vi "BUILD_uninstall tag bus.vi"() -> ()   [LabVIEW 2013]
panel:
  out "error out":errorcluster
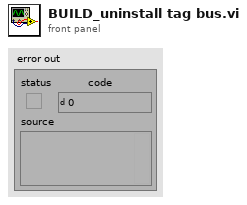
[diagram p1: front panel]
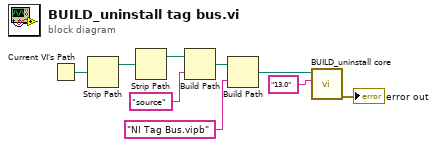
[diagram p0: block diagram]
diagram:
  n1 = Current VI's Path() -> (path=w9:path)
  n2 = Strip Path(path=w9) -> (stripped path=w8:path)  [unwired: 1 out]
  n3 = Strip Path(path=w8) -> (stripped path=w6:path)  [unwired: 1 out]
  n4 = Build Path(base path=w6, name or relative path="source") -> (appended path=w4:path)
  n5 = Build Path(base path=w4, name or relative path="NI Tag Bus.vipb") -> (appended path=w1:path)
  n6 = call "BUILD_uninstall core.vi"("LabVIEW Version"="13.0", "appended path"=w1) -> ("error out"=→"error out":errorcluster)  [unwired: 9 in]
